vi "Create.vi"(8 "error in (no error)":errorcluster, 10 "Port Config (115200 8N1)":T1={"Baud (115200)"=115200, "Data Bits (8)"=8, "Stop Bits (1)"=10, "Flow Control"=0, "Use LineTerm?"=FALSE, "LineTerm (\\n)"="\n", "Timeout ms (10000)"=10000, "Parity (None)"=enum."None"} {"Flow Control" items=["None", "XON/XOFF", "RTS/CTS", "XON/XOFF & RTS/CTS", "DTR/DSR", "XON/XOFF & DTR/DSR"]; "Stop Bits (1)" items=["1.0"=10, "1.5"=15, "2.0"=20]}, 11 "Serial Port":refnum<visa-resource-name>) -> (0 "error out":errorcluster, 3 "SerialResource out":refnum<class "SerialResource.lvclass">)   [LabVIEW 2020, in "PicoG-Core.lvlib" / "SerialResource.lvclass"]
uses:
  SerialResource.lvclass
  SerialResource.lvclass/SerialResource.ctl
  <vilib>/IlluminatedG/IG Serial Stream/Stream-Serial/Serial Client/Serial Client.lvclass
  <vilib>/IlluminatedG/IG Serial Stream/Stream-Serial/Serial Client/Stop Bits.ctl
  <vilib>/IlluminatedG/IG Serial Stream/Stream-Serial/Serial Client/Flow Control.ctl
  <vilib>/IlluminatedG/IG Serial Stream/Stream-Serial/Serial Client/Parity.ctl
  <vilib>/IlluminatedG/IG Serial Stream/Stream-Serial/Serial Client/Port Config.ctl
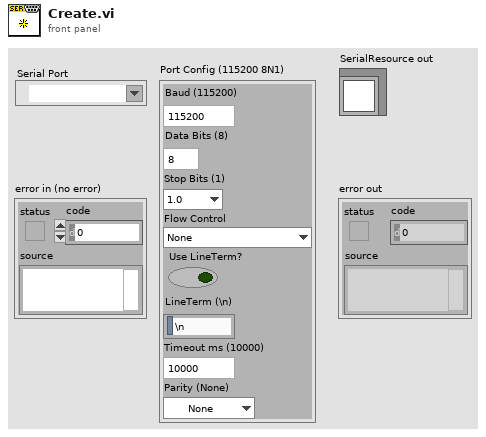
[diagram p1: front panel]
types:
  T1 = typedef "Stream-Serial.lvlib/Serial Client.lvclass/Port Config.ctl" = cluster{"Baud (115200)":u32, "Data Bits (8)":u8, "Stop Bits (1)":T2, "Flow Control":T3, "Use LineTerm?":bool, "LineTerm (\\n)":string, "Timeout ms (10000)":i32, "Parity (None)":T4}
  T2 = typedef "Stream-Serial.lvlib/Serial Client.lvclass/Stop Bits.ctl" = u16
  T3 = typedef "Stream-Serial.lvlib/Serial Client.lvclass/Flow Control.ctl" = u16
  T4 = typedef "Stream-Serial.lvlib/Serial Client.lvclass/Parity.ctl" = enum16{"None", "Odd", "Even", "Mark", "Space"}
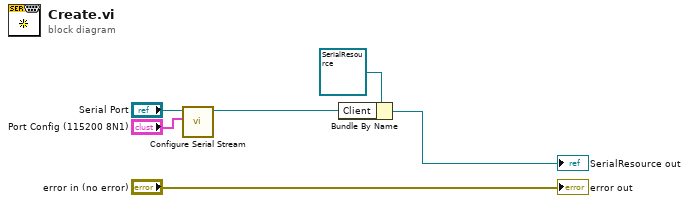
[diagram p0: block diagram]
diagram:
  n1 = call <vilib>:"Configure Serial Stream.vi"("Port Config (115200 8N1)"="Port Config (115200 8N1)", "Serial Port"="Serial Port") -> ("Serial Client out"=w1:refnum<class "Serial Client.lvclass">)  [unwired: 8 in, 1 out]
  n2 = Bundle By Name(cluster=refnum<class "SerialResource.lvclass"> refnum ("SerialResource in"), "Client"=w1) -> (→"SerialResource out":refnum<class "SerialResource.lvclass">)
  "error out" <- "error in (no error)"
